vi "terminate.vi"(8 "error in (no error)":errorcluster, 11 "PointCollection in":refnum<class "PointCollection.lvclass">) -> (0 "error out":errorcluster, 2 "point array":dbl[][](array[numeric]), 3 "PointCollection out":refnum<class "PointCollection.lvclass">)   [LabVIEW 2010, in "PointCollection.lvclass"]
uses:
  PointCollection.lvclass
  PointCollection.lvclass/PointCollection.ctl
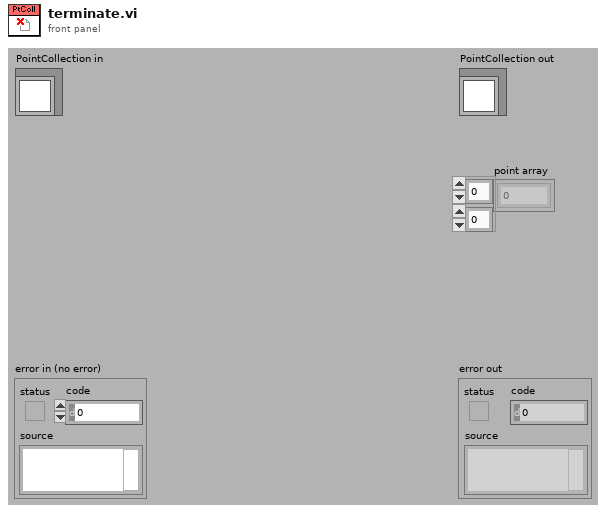
[diagram p1: front panel]
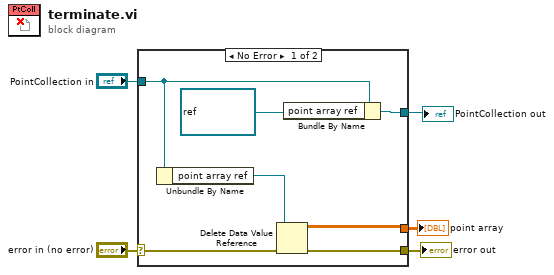
[diagram p0: block diagram]
diagram:
  n1 = case shown="No Error" "error in (no error)" {
    selector: "error in (no error)" -> [w6 w14]
    tunnel: [w12 w14] -> w4
    tunnel: [w9 w13] -> w2
    tunnel: "PointCollection in" -> [w10 w13]
    tunnel: [w8 _] -> w1
    frame No Error {
      n2 = Unbundle By Name(w10) -> ("point array ref"=w7:refnum<data-value>)
      n3 = Delete Data Value Reference(data value reference=w7, error in=w6) -> (data value=w8:dbl[][], error out=w12:errorcluster)
      n4 = Bundle By Name(cluster=w10, "point array ref"=refnum<data-value> refnum ("data value reference")) -> (w9:refnum<class "PointCollection.lvclass">)
    }
    frame Error {
    }
  }
  "error out" <- w4
  "PointCollection out" <- w2
  "point array" <- w1
